vi "3.2-What.vi"() -> (1 "Heartbeat":bool)   [LabVIEW 2010]
uses:
  3.0-Global.vi
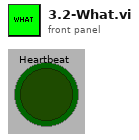
[diagram p1: front panel]
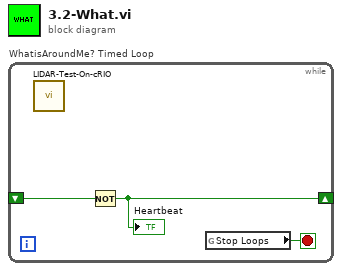
[diagram p0: block diagram]
diagram:
  n1 = while "WhatisAroundMe? Timed Loop" {
    shift-right: [w2] -> _
    shift-left: _ -> [w3]
    stop <- w1 stop-if-true
    n2 = call "LIDAR-Test-On-cRIO.vi"() -> ()  [unwired: 12 in]
    n3 = Not(x=w3) -> (.not. x?=w2:bool)
    "Heartbeat" <- w2
    n4 = global read "3.0-Global.vi" "Stop Loops"() -> (w1:bool)
  }
